vi "ex_CreateBackupName.vi"(4 "original name":path) -> (1 "backup name":path)   [LabVIEW 2017]
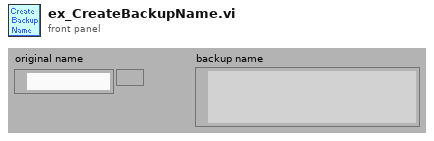
[diagram p1: front panel]
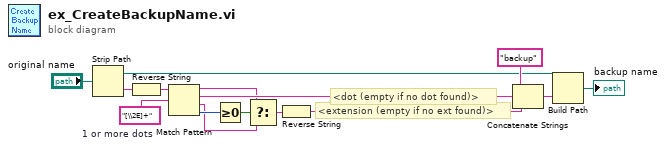
[diagram p0: block diagram]
diagram:
  w14 = "[\\2E]+"  # 1 or more dots
  # "<dot (empty if no dot found)>"
  # "<extension (empty if no ext found)>"
  n1 = Strip Path(path="original name") -> (stripped path=w6:path, name=w9:string)
  n2 = Reverse String(1:w9) -> (0:w15:string)
  n3 = Match Pattern(string=w15, regular expression=w14) -> (before substring=w3:string, match substring=w12:string, after substring=w2:string, offset past match=w4:i32)  [unwired: 1 out]
  n4 = Greater Or Equal To 0?(x=w4) -> (x >= 0?=w5:bool)
  n5 = Select(t=w3, s=w5, f=w2) -> (s? t:f=w1:string)
  n6 = Reverse String(1:w1) -> (0:w13:string)
  n7 = Concatenate Strings("backup" ("Substring"), w12, w13) -> (w8:string)
  n8 = Build Path(base path=w6, name or relative path=w8) -> (appended path=→"backup name":path)
